vi "test Import Configuration File (Non Default Attributes).vi"(8 "error in (no error)":errorcluster, 11 "TestCase in":refnum<class "AIM ARINC 664 Import.lvclass">) -> (0 "error out":errorcluster, 3 "TestCase out":refnum<class "AIM ARINC 664 Import.lvclass">)   [LabVIEW 2020, in "AIM ARINC 664 Import.lvclass"]
uses:
  AIM ARINC 664 Import.lvclass
  Import/_typedefs/Board Top Level Configuration.ctl
  Import/_typedefs/board_setup.ctl
  Import/_typedefs/port_configuration.ctl
  Import/_typedefs/port_setup.ctl
  Import/_typedefs/session_tx_generic.ctl
  Import/_typedefs/tx_generic_setup.ctl
  Import/_typedefs/frame_tx_generic.ctl
  Import/_typedefs/frame_tx_generic_seqNumberInit.ctl
  Import/_typedefs/frame_tx_generic_seqNumberOffset.ctl
  Import/_typedefs/frame_parameter.ctl
  Import/_typedefs/frame_parameter_definition.ctl
  Shared/Encoding (Arinc664).ctl
  Import/_typedefs/port_tx_udp_comm.ctl
  Import/_typedefs/port_tx_udp_sap.ctl
  Import/_typedefs/rx_udp_setup.ctl
  Import/_typedefs/port_rx_udp_comm.ctl
  Import/_typedefs/port_rx_udp_sap.ctl
  <vilib>/addons/_JKI Toolkits/VI Tester/TestCase.llb/TestCase.lvclass
  <userlib>/_OpenG.lib/appcontrol/appcontrol.llb/openg_application_control.lvlib
  <vilib>/NI/VeriStand Custom Device Testing Tools/VeriStandTestUtilities/VeriStandTestUtilities.lvlib
  Import/AIM ARINC 664 Import.lvlib
  C:/Program Files/National Instruments/LabVIEW 2024/vi.lib/addons/_JKI Toolkits/VI Tester/TestCase.llb/TestCase.lvclass
panel:
  out "x = y? 2":bool[](array[boolean])
  out "logical AND 6":bool
  out "index of element":i32[](array[numeric])
  out "size(s)":i32
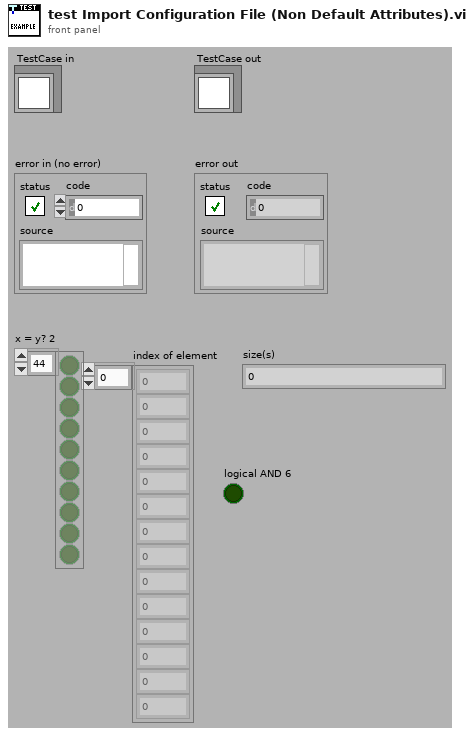
[diagram p1: front panel]
types:
  T1 = typedef "AIM ARINC 664 Import.lvlib/Board Top Level Configuration.ctl" = cluster{"boardSetup":T2, "portConfiguration":T3[]}
  T2 = typedef "AIM ARINC 664 Import.lvlib/board_setup.ctl" = cluster{"boardId":u32, "portSpeed":u32, "portConfig":u32}
  T3 = typedef "AIM ARINC 664 Import.lvlib/port_configuration.ctl" = cluster{"portSetup":T4, "Tx_Generic":T5[], "Rx_Monitor":cluster{"DefaultCronoMode":u32, "GlbMonBufferSizeIn":u32, "CaptureMode":u32, "MaxFileSizeMB":u32, "Strobe":u32, "TriggerPosition":u32}[], "Tx_UDP":cluster{"tx_udp_setup":cluster{"VlId":i32, "Bag":i32, "NetSelect":u32, "domainID":u8, "sideID":u8, "locationID":u8, "interfaceID":u8, "NumOfSubVl":u16, "Skew":u32, "MaxFrameLength":u32, "FrameBufferSize":u32}, "commPorts":T13[], "sapPorts":T14[]}[], "Rx_UDP":cluster{"Tx_UDP":T15, "commPorts":T16[], "sapPorts":T17[]}[]}
  T4 = typedef "AIM ARINC 664 Import.lvlib/port_setup.ctl" = cluster{"port Id":u32, "redundant":bool}
  T5 = typedef "AIM ARINC 664 Import.lvlib/session_tx_generic.ctl" = cluster{"tx_generic_setup":T6, "Frame Headers":T7[]}
  T6 = typedef "AIM ARINC 664 Import.lvlib/tx_generic_setup.ctl" = cluster{"QueueSizeIn":u32, "Count":i32, "StartMode":i32}
  T7 = typedef "AIM ARINC 664 Import.lvlib/frame_tx_generic.ctl" = cluster{"FrameID":string, "PayloadID":string, "Frame header":cluster{"FrameStartMode":i32, "InterFrameGap":i32, "PacketGroupWaitTime":i32, "NetSelect":u32, "PayloadBufferMode":i32, "PayloadGenerationMode":i32, "PhysErrorInjection":i32, "PreambleCount":i32, "SequenceNumberInit":T8, "SequenceNumberOffset":T9, "Skew":i32}, "Parameters":T10[]}
  T8 = typedef "AIM ARINC 664 Import.lvlib/frame_tx_generic_seqNumberInit.ctl" = i32
  T9 = typedef "AIM ARINC 664 Import.lvlib/frame_tx_generic_seqNumberOffset.ctl" = i32
  T10 = typedef "AIM ARINC 664 Import.lvlib/frame_parameter.ctl" = cluster{"name":string, "default value":dbl, "unit":string, "Parameter":T11}
  T11 = typedef "AIM ARINC 664 Import.lvlib/frame_parameter_definition.ctl" = cluster{"start index":i32, "size":i32, "encoding":T12, "signed":bool, "scale multiplier":dbl, "scale offset":dbl}
  T12 = typedef "Encoding (Arinc664).ctl" = u16
  T13 = typedef "AIM ARINC 664 Import.lvlib/port_tx_udp_comm.ctl" = cluster{"PayloadID":string, "partitionID":u8, "UdpSrcPort":u16, "UdpDstPort":u16, "PortType":enum16{"FDX_UDP_SAMPLING", "FDX_UDP_QUEUING"}, "SubVIId":u32, "UdpNumBufMessages":u32, "UdpMaxMessageSize":u32, "UdpSamplingRate":u32, "Parameters":T10[]}
  T14 = typedef "AIM ARINC 664 Import.lvlib/port_tx_udp_sap.ctl" = cluster{"PayloadID":string, "SubVlId":u8, "UdpSrcPort":u16, "UdpNumBufMessages":u32, "UdpMaxMessageSize":u32, "partitionID":u8, "domainID":u8, "sideID":u8, "locationID":u8, "interfaceID":u8, "Parameters":T10[]}
  T15 = typedef "AIM ARINC 664 Import.lvlib/rx_udp_setup.ctl" = cluster{"VerificationMode":u32, "Bag":u32, "Jitter":u32, "MaxFrameLength":u32, "MaxSkew":u32, "VLBufSize":u32, "FilterMode":u32, "FilterPosition":u32, "Padding":u32, "FilterMask":u32, "FilterData":u32, "MinFrameLength":u32, "VlId":u16, "VLRange":u32}
  T16 = typedef "AIM ARINC 664 Import.lvlib/port_rx_udp_comm.ctl" = cluster{"PayloadID":string, "domainID":u8, "sideID":u8, "locationID":u8, "partitionID":u8, "UdpSrcPort":u16, "UdpDstPort":u16, "PortType":enum16{"FDX_UDP_SAMPLING", "FDX_UDP_QUEUING"}, "SubVIId":u32, "UdpNumBufMessages":u32, "UdpMaxMessageSize":u32, "UdpSamplingRate":u32, "Parameters":T10[]}
  T17 = typedef "AIM ARINC 664 Import.lvlib/port_rx_udp_sap.ctl" = cluster{"PayloadID":string, "UdpDstPort":u16, "UdpNumBufMessages":u32, "UdpMaxMessageSize":u32, "Parameters":T10[]}
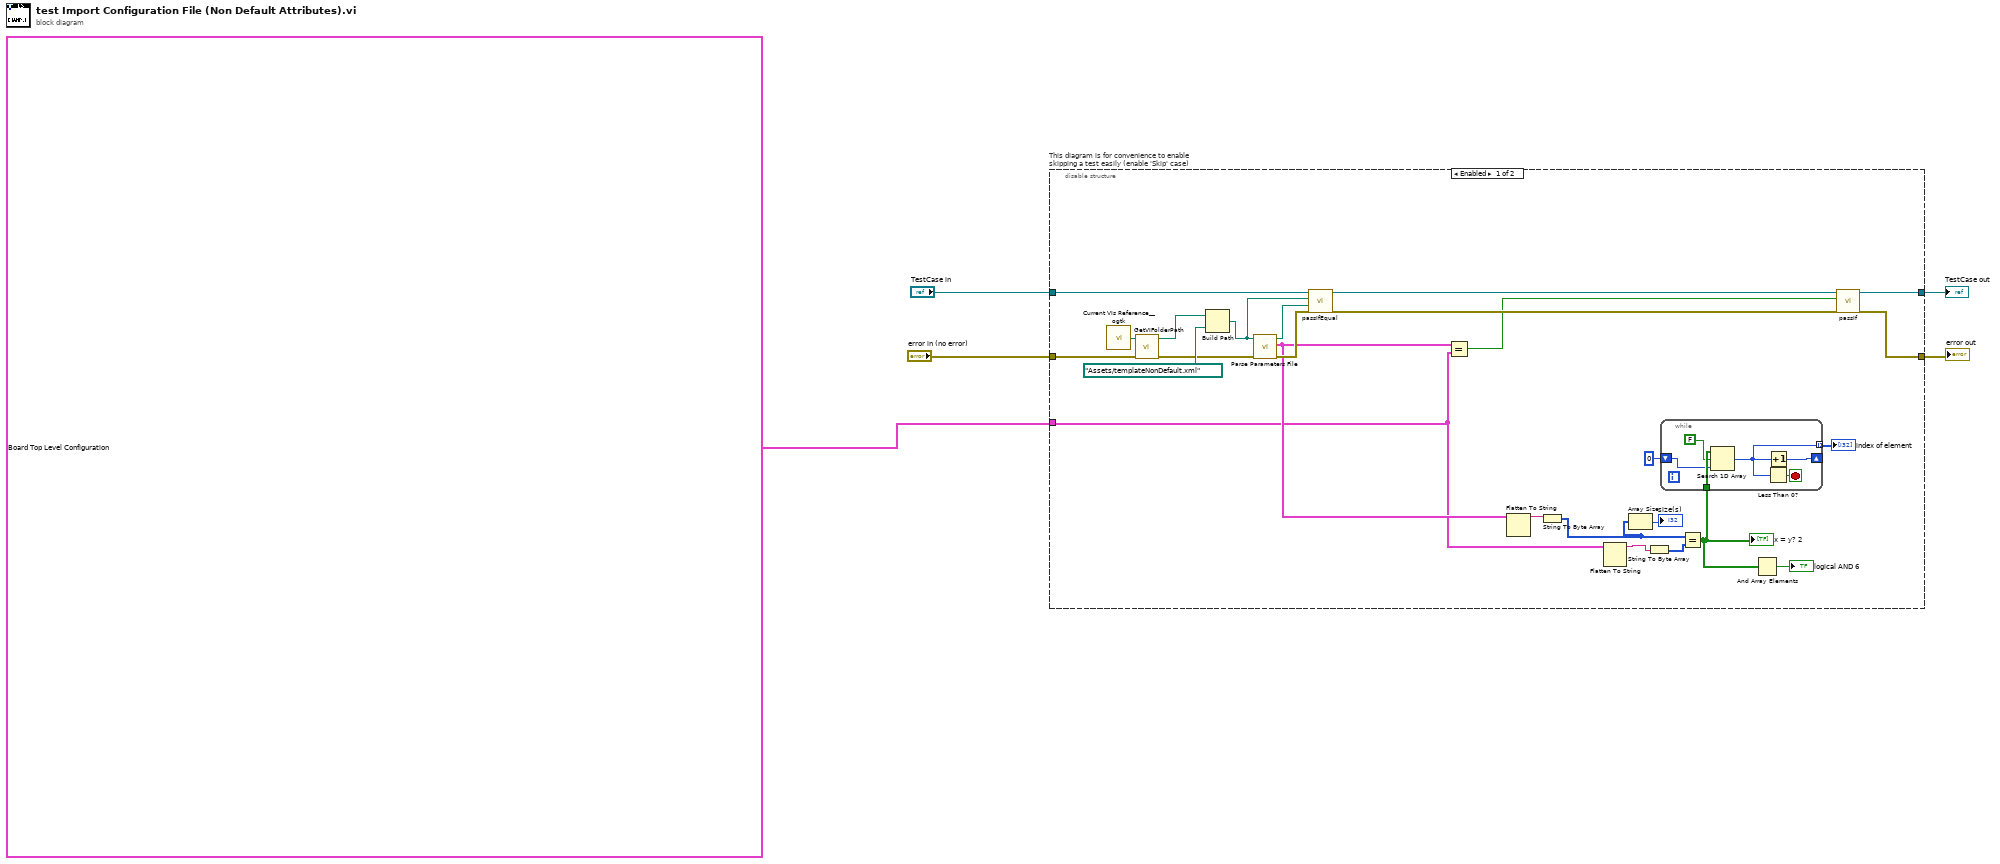
[diagram p0: block diagram]
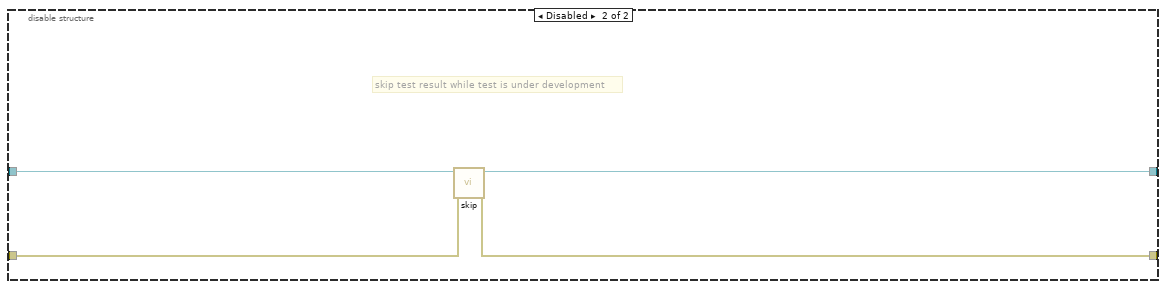
[diagram p2: hidden frame]
diagram:
  n1 = disable-structure "This diagram is for convenience to enable skipping a test easily (enable 'Skip' case)" shown="Enabled" {
    disable-tunnel: "TestCase in" -> [w23 w40]
    disable-tunnel: [w25 w38] -> w2
    disable-tunnel: [w24 w39] -> w4
    disable-tunnel: "error in (no error)" -> [w28 w37]
    disable-tunnel: T1 {"boardSetup"={"boardId"=1, "portSpeed"=1, "portConfig"=1}, "portConfiguration"=[{"portSetup"={"port Id"=2, "redundant"=FALSE}, "Tx_Generic"=[{"tx_generic_setup"={"QueueSizeIn"=3, "Count"=6, "StartMode"=3}, "Frame Headers"=[{"FrameID"="", "PayloadID"="0", "Frame header"={"FrameStartMode"=1, "InterFrameGap"=0, "PacketGroupWaitTime"=0, "NetSelect"=3, "PayloadBufferMode"=0, "PayloadGenerationMode"=0, "PhysErrorInjection"=0, "PreambleCount"=7, "SequenceNumberInit"=65535, "SequenceNumberOffset"=65535, "Skew"=0}, "Parameters"=[]}]}], "Rx_Monitor"=[{"DefaultCronoMode"=2, "GlbMonBufferSizeIn"=2, "CaptureMode"=3, "MaxFileSizeMB"=4, "Strobe"=2, "TriggerPosition"=3}], "Tx_UDP"=[], "Rx_UDP"=[]}, {"portSetup"={"port Id"=3, "redundant"=FALSE}, "Tx_Generic"=[], "Rx_Monitor"=[], "Tx_UDP"=[{"tx_udp_setup"={"VlId"=4, "Bag"=2, "NetSelect"=4, "domainID"=1, "sideID"=12, "locationID"=2, "interfaceID"=2, "NumOfSubVl"=3, "Skew"=5, "MaxFrameLength"=3, "FrameBufferSize"=1}, "commPorts"=[{"PayloadID"="TxUDP", "partitionID"=123, "UdpSrcPort"=444, "UdpDstPort"=22, "PortType"=enum."FDX_UDP_QUEUING", "SubVIId"=233, "UdpNumBufMessages"=2425, "UdpMaxMessageSize"=11, "UdpSamplingRate"=344, "Parameters"=[{"name"="Param 0", "default value"=1.0, "unit"="x", "Parameter"={"start index"=2, "size"=29, "encoding"=1, "signed"=TRUE, "scale multiplier"=3.14, "scale offset"=2.0}}, {"name"="Param 1", "default value"=1.0, "unit"="x", "Parameter"={"start index"=2, "size"=29, "encoding"=1, "signed"=TRUE, "scale multiplier"=3.14, "scale offset"=2.0}}, {"name"="Param 2", "default value"=1.0, "unit"="x", "Parameter"={"start index"=2, "size"=29, "encoding"=1, "signed"=TRUE, "scale multiplier"=3.14, "scale offset"=2.0}}]}], "sapPorts"=[{"PayloadID"="TxSAP", "SubVlId"=4, "UdpSrcPort"=123, "UdpNumBufMessages"=134, "UdpMaxMessageSize"=4, "partitionID"=6, "domainID"=2, "sideID"=8, "locationID"=5, "interfaceID"=4, "Parameters"=[{"name"="Param 0", "default value"=1.0, "unit"="x", "Parameter"={"start index"=2, "size"=29, "encoding"=1, "signed"=TRUE, "scale multiplier"=3.14, "scale offset"=2.0}}, {"name"="Param 1", "default value"=1.0, "unit"="x", "Parameter"={"start index"=2, "size"=29, "encoding"=1, "signed"=TRUE, "scale multiplier"=3.14, "scale offset"=2.0}}, {"name"="Param 2", "default value"=1.0, "unit"="x", "Parameter"={"start index"=2, "size"=29, "encoding"=1, "signed"=TRUE, "scale multiplier"=3.14, "scale offset"=2.0}}]}]}], "Rx_UDP"=[{"Tx_UDP"={"VerificationMode"=4, "Bag"=2, "Jitter"=2, "MaxFrameLength"=8, "MaxSkew"=6, "VLBufSize"=44, "FilterMode"=1, "FilterPosition"=5, "Padding"=0, "FilterMask"=6, "FilterData"=4, "MinFrameLength"=46, "VlId"=34, "VLRange"=33}, "commPorts"=[{"PayloadID"="RxUDP", "domainID"=1, "sideID"=4, "locationID"=3, "partitionID"=4, "UdpSrcPort"=245, "UdpDstPort"=4, "PortType"=enum."FDX_UDP_QUEUING", "SubVIId"=1, "UdpNumBufMessages"=8, "UdpMaxMessageSize"=6, "UdpSamplingRate"=0, "Parameters"=[{"name"="Param 0", "default value"=0.0, "unit"="", "Parameter"={"start index"=0, "size"=0, "encoding"=0, "signed"=FALSE, "scale multiplier"=0.0, "scale offset"=0.0}}, {"name"="Param 1", "default value"=0.0, "unit"="", "Parameter"={"start index"=0, "size"=0, "encoding"=0, "signed"=FALSE, "scale multiplier"=0.0, "scale offset"=0.0}}]}], "sapPorts"=[{"PayloadID"="RxSAP", "UdpDstPort"=1, "UdpNumBufMessages"=3, "UdpMaxMessageSize"=2, "Parameters"=[{"name"="Param 0", "default value"=0.0, "unit"="", "Parameter"={"start index"=0, "size"=0, "encoding"=0, "signed"=FALSE, "scale multiplier"=0.0, "scale offset"=0.0}}, {"name"="Param 1", "default value"=0.0, "unit"="", "Parameter"={"start index"=0, "size"=0, "encoding"=0, "signed"=FALSE, "scale multiplier"=0.0, "scale offset"=0.0}}]}]}]}]} ("board configuration out") -> [w6 _]
    frame Enabled {
      n2 = call <userlib>:"Current VIs Reference__ogtk.vi"() -> ("Current VI's reference"=w30:refnum<vi>)  [unwired: 5 in]
      n3 = call <vilib>:"GetVIFolderPath.vi"("error in (no error)"=w28, "VI Reference in"=w30) -> ("error out"=w26:errorcluster, "VI Folder Path out"=w29:path)  [unwired: 8 in]
      n4 = Build Path(base path=w29, name or relative path=path "Assets/templateNonDefault.xml") -> (appended path=w20:path)
      n5 = call "Parse Parameters File.vi"("error in"=w26, "path to XML document"=w20) -> ("error out"=w21:errorcluster, "board configuration out"=w7:T1, "path to XML document out"=w19:path)  [unwired: 7 in]
      n6 = call-dynamic "passIfEqual.vi"("error in (no error)"=w21, "y"=w19, "x"=w20, "TestCase in"=w23) -> ("error out"=w18:errorcluster, "TestCase out"=w22:refnum<class "AIM ARINC 664 Import.lvclass">)  [unwired: 6 in]
      n7 = Equal?(x=w7, y=w6) -> (x = y?=w17:bool)
      n8 = Flatten To String(anything=w7) -> (data string=w16:string)  [unwired: 3 in, 2 out]
      n9 = String To Byte Array(string=w16) -> (unsigned byte array=w11:u8[])
      n10 = Flatten To String(anything=w6) -> (data string=w15:string)  [unwired: 3 in, 2 out]
      n11 = Array Size(array=w11) -> (size(s)=→"size(s)":i32)
      n12 = String To Byte Array(string=w15) -> (unsigned byte array=w14:u8[])
      n13 = Equal?(x=w11, y=w14) -> (x = y?=w12:bool[])
      "x = y? 2" <- w12
      n14 = while {
        tunnel: w12 -> [w36]
        tunnel: [w33] -> w9 mode=indexing
        shift-right: [w31] -> _
        shift-left: 0 ("index of element") -> [w32]
        stop <- w34 stop-if-true
        n15 = Search 1D Array(1D array=w36, element=FALSE ("logical AND 6"), start index (0)=w32) -> (index of element=w33:i32)
        n16 = Less Than 0?(x=w33) -> (x < 0?=w34:bool)
        n17 = Increment(x=w33) -> (x+1=w31:i32)
      }
      "index of element" <- w9
      n18 = And Array Elements(Boolean array=w12) -> (logical AND=→"logical AND 6":bool)
      n19 = call-dynamic "passIf.vi"("error in (no error)"=w18, "pass"=w17, "TestCase in"=w22) -> ("error out"=w24:errorcluster, "TestCase out"=w25:refnum<class "AIM ARINC 664 Import.lvclass">)  [unwired: 7 in]
    }
    frame Disabled {
      # "skip test result while test is under development"
      n20 = call <vilib>:"skip.vi"("error in (no error)"=w37, "TestCase in"=w40) -> ("error out"=w39:errorcluster, "TestCase out"=w38:refnum<class "AIM ARINC 664 Import.lvclass">)  [unwired: 8 in]
    }
  }
  "error out" <- w4
  "TestCase out" <- w2
